vi "WPI_GetSetVariantRefNum.vi"(6 "Test Mode Only":bool, 7 "prefix":string, 8 "error in (no error)":errorcluster, 9 "Operation":T1, 10 "refnum name":string, 11 "DevRef":variant) -> (0 "error out":errorcluster, 2 "names":string[](array[string]), 3 "DevRef":variant)   [LabVIEW 2025]
doc: "Sets a reference into a registry, gets a reference from a registry, or deletes a reference from a registry. The reference is accessed by name, and can be given any unique name.\n\nThis software is licensed. Open the labview\\readme\\WPI Robotics Library Open Source License.txt file for more information."
uses:
  <vilib>/Rock Robotics/WPI/Utilities/Refnum Registry Operation.ctl
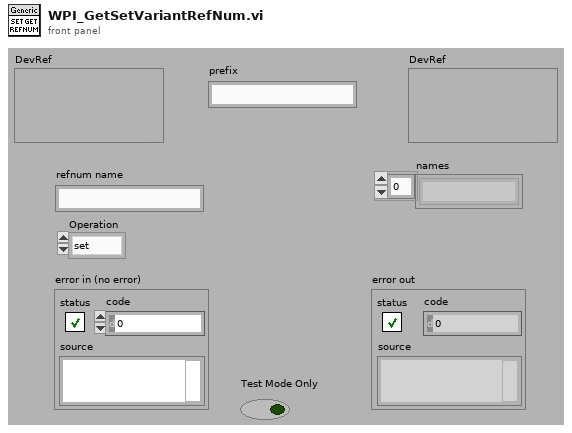
[diagram p1: front panel]
types:
  T1 = typedef "Refnum Registry Operation.ctl" = enum16{"set", "get", "delete", "get all names", "read name"}
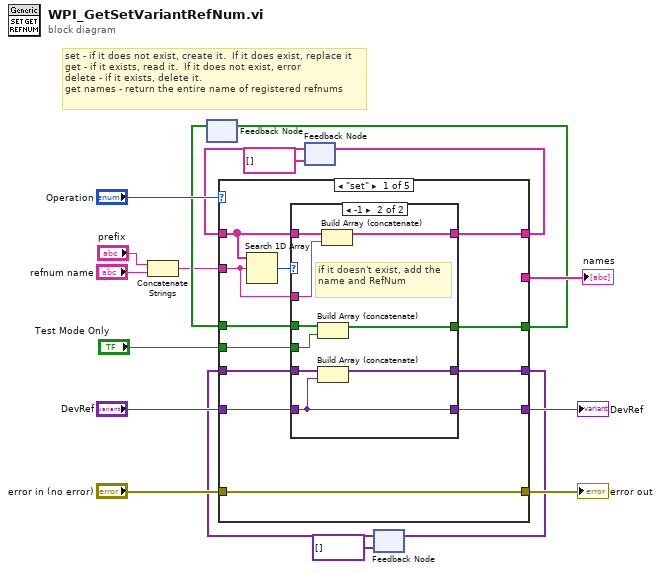
[diagram p0: block diagram]
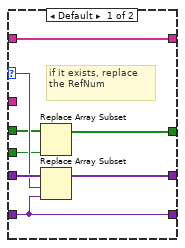
[diagram p2: hidden frame]
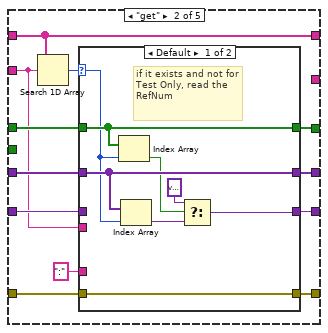
[diagram p3: hidden frame]
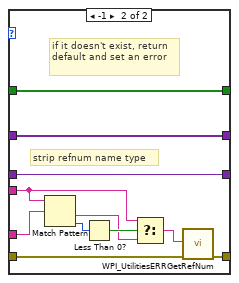
[diagram p4: hidden frame]
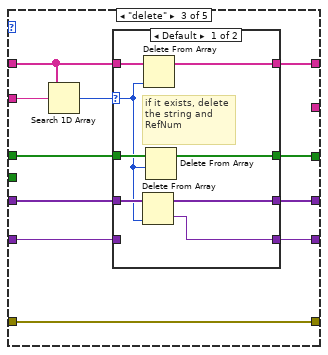
[diagram p5: hidden frame]
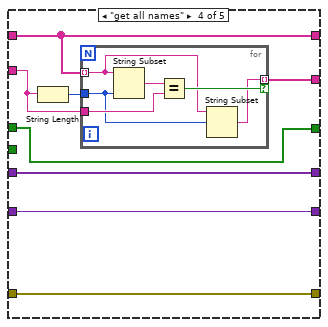
[diagram p7: hidden frame]
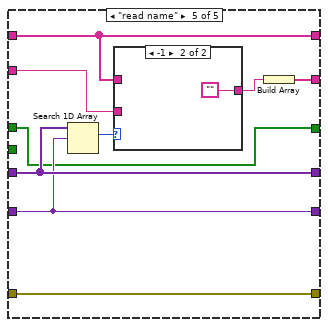
[diagram p8: hidden frame]
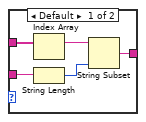
[diagram p9: hidden frame]
diagram:
  # "set - if it does not exist, create it.  If it does exist, replace it\nget - if it exists, read it.  If it does not exist, error\ndelete - if it exists, delete it.\nget names - return the entire name of registered refnums"
  n1 = Concatenate Strings("prefix", "refnum name") -> (w1:string)
  n2 = feedback #1() -> (w6:bool[])  [unwired: 1 in]
  n3 = feedback #2(string[] []) -> (w9:string[])
  n4 = feedback #3(variant[] []) -> (w11:variant[])
  n5 = case shown="\"set\"" "Operation" {
    tunnel: "DevRef" -> [w25 w57 w84 w108 w122]
    tunnel: [w24 w56 w83 w109 w123] -> w12
    tunnel: w11 -> [w26 w58 w85 w109 w123]
    tunnel: [w23 w55 w82 w108 w122] -> w17
    tunnel: [w30 w54 w89 w106 w117] -> w10
    tunnel: w9 -> [w29 w54 w88 w106 w117]
    tunnel: w1 -> [w27 w49 w86 w104 w116]
    tunnel: [w22 w52 w81 w107 w124] -> w15
    tunnel: "error in (no error)" -> [w22 w53 w81 w107 w124]
    tunnel: [_ _ _ w103 w121] -> w13
    tunnel: w6 -> [w21 w51 w80 w102 w120]
    tunnel: [w20 w50 w79 w102 w120] -> w5
    tunnel: "Test Mode Only" -> [w19 _ _ _ _]
    frame "set" {
      n6 = Search 1D Array(1D array=w29, element=w27) -> (index of element=w28:i32)  [unwired: 1 out]
      n7 = case shown="-1" w28 {
        selector: w28 -> [w36 _]
        tunnel: [w38 w47] -> w30
        tunnel: w29 -> [w38 w46]
        tunnel: w27 -> [_ w45]
        tunnel: w26 -> [w37 w44]
        tunnel: w25 -> [w34 w42]
        tunnel: [w35 w43] -> w24
        tunnel: [w34 w42] -> w23
        tunnel: w21 -> [w33 w41]
        tunnel: [w32 w39] -> w20
        tunnel: w19 -> [w31 w40]
        frame Default {
          # "if it exists, replace the RefNum"
          n8 = Replace Array Subset(array=w33, new element=w31) -> (w32:bool[])  [unwired: 1 in]
          n9 = Replace Array Subset(array=w37, new element=w34, index=w36) -> (w35:variant[])
        }
        frame -1 {
          # "if it doesn't exist, add the name and RefNum"
          n10 = Build Array (concatenate)(w41, w40) -> (w39:bool[])
          n11 = Build Array (concatenate)(w44, w42) -> (w43:variant[])
          n12 = Build Array (concatenate)(w46, w45) -> (w47:string[])
        }
      }
    }
    frame "get" {
      n13 = Search 1D Array(1D array=w54, element=w49) -> (index of element=w59:i32)  [unwired: 1 out]
      n14 = case shown="Default" w59 {
        selector: w59 -> [w64 _]
        tunnel: w58 -> [w67 w78]
        tunnel: w57 -> [_ w69]
        tunnel: [w67 w78] -> w56
        tunnel: [w63 w69] -> w55
        tunnel: w53 -> [w66 w76]
        tunnel: [w66 w77] -> w52
        tunnel: w51 -> [w65 w75]
        tunnel: [w65 w75] -> w50
        tunnel: w49 -> [_ w71]
        tunnel: ":" ("regular expression") -> [_ w68]
        frame Default {
          # "if it exists and not for Test Only, read the RefNum"
          n15 = Index Array(array=w65, index=w64) -> (element=w62:bool)
          n16 = Index Array(array=w67, index=w64) -> (element=w60:variant)
          n17 = Select(t=variant ("f"), s=w62, f=w60) -> (s? t:f=w63:variant)
        }
        frame -1 {
          # "strip refnum name type"
          # "if it doesn't exist, return default and set an error"
          n18 = Match Pattern(string=w71, regular expression=w68) -> (after substring=w72:string, offset past match=w74:i32)  [unwired: 1 in, 2 out]
          n19 = Less Than 0?(x=w74) -> (x < 0?=w73:bool)
          n20 = Select(t=w71, s=w73, f=w72) -> (s? t:f=w70:string)
          n21 = call <vilib>:"WPI_UtilitiesERRGetRefNum.vi"("error in (no error)"=w76, "unfound refnum name"=w70) -> ("ERRGetRefNum"=w77:errorcluster)  [unwired: 9 out]
        }
      }
    }
    frame "delete" {
      n22 = Search 1D Array(1D array=w88, element=w86) -> (index of element=w87:i32)  [unwired: 1 out]
      n23 = case shown="Default" w87 {
        selector: w87 -> [w91 _]
        tunnel: [w93 w100] -> w89
        tunnel: w88 -> [w94 w100]
        tunnel: w85 -> [w97 w99]
        tunnel: w84 -> [_ w101]
        tunnel: [w96 w99] -> w83
        tunnel: [w95 w101] -> w82
        tunnel: w80 -> [w92 w98]
        tunnel: [w90 w98] -> w79
        frame Default {
          # "if it exists, delete the string and RefNum"
          n24 = Delete From Array(array=w97, index=w91) -> (deleted portion=w95:variant, array with subset deleted=w96:variant[])  [unwired: 1 in]
          n25 = Delete From Array(array=w94, index=w91) -> (array with subset deleted=w93:string[])  [unwired: 1 in, 1 out]
          n26 = Delete From Array(array=w92, length=w91) -> (array with subset deleted=w90:bool[])  [unwired: 1 in, 1 out]
        }
        frame -1 {
          # "if it doesn't exist, do nothing"
        }
      }
    }
    frame "get all names" {
      n27 = String Length(string=w104) -> (length=w105:i32)
      n28 = for {
        tunnel: w106 -> [w111] mode=indexing
        tunnel: w105 -> [w112]
        tunnel: w104 -> [w113]
        tunnel: [w110] -> w103 mode=indexing if=w114
        n29 = String Subset(string=w111, length (rest)=w112) -> (substring=w115:string)  [unwired: 1 in]
        n30 = Equal?(x=w115, y=w113) -> (x = y?=w114:bool)
        n31 = String Subset(string=w111, offset (0)=w112) -> (substring=w110:string)  [unwired: 1 in]
      }
    }
    frame "read name" {
      n32 = Search 1D Array(1D array=w123, element=w122) -> (index of element=w119:i32)  [unwired: 1 in]
      n33 = case shown="-1" w119 {
        tunnel: [w125 ""] -> w118
        tunnel: w117 -> [w129 _]
        tunnel: w116 -> [w128 _]
        frame Default {
          n34 = Index Array(array=w129) -> (element=w126:string)  [unwired: 1 in]
          n35 = String Length(string=w128) -> (length=w127:i32)
          n36 = String Subset(string=w126, length (rest)=w127) -> (substring=w125:string)  [unwired: 1 in]
        }
        frame -1 {
        }
      }
      n37 = Build Array(w118) -> (w121:string[])
    }
  }
  "error out" <- w15
  "DevRef" <- w17
  "names" <- w13
  n38 = feedback-in #1(w5) -> ()
  n39 = feedback-in #2(w10) -> ()
  n40 = feedback-in #3(w12) -> ()
